vi "Query Operation Complete.vi"(8 "error in (no error)":errorcluster, 11 "VISA resource name":refnum<visa-resource-name>) -> (0 "error out":errorcluster, 2 "Operation Status":u8, 3 "VISA resource name out":refnum<visa-resource-name>)   [LabVIEW 2018, in "LTB-1.lvlib" / "3150.lvlib"]
doc: "Allows the synchronization between the instrument and an external controller by reading the Output Queue or by waiting for a service request on the Message Available (MAV) bit in the Status Byte Register."
uses:
  3150.lvlib
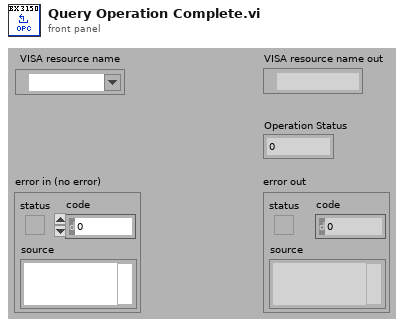
[diagram p1: front panel]
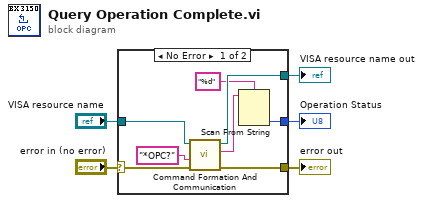
[diagram p0: block diagram]
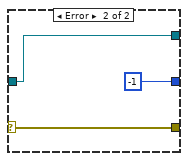
[diagram p2: hidden frame]
diagram:
  n1 = case shown="No Error" "error in (no error)" {
    selector: "error in (no error)" -> [w13 w16]
    tunnel: [w12 w16] -> w1
    tunnel: [w11 w15] -> w3
    tunnel: "VISA resource name" -> [w10 w15]
    tunnel: [w7 -1] -> w5
    frame No Error {
      n2 = call "Command Formation And Communication.vi"("error in (no error)"=w13, "Command"="*OPC?", "VISA resource name"=w10) -> ("error out"=w12:errorcluster, "Response"=w8:string, "VISA resource name out"=w11:refnum<visa-resource-name>)  [unwired: 1 in, 5 out]
      n3 = Scan From String(format string="%d", input string=w8) -> (output 1=w7:i32)  [unwired: 2 in, 4 out]
    }
    frame Error {
    }
  }
  "Operation Status" <- w5
  "VISA resource name out" <- w3
  "error out" <- w1
